vi "4031V2Project.vi"() -> ()   [LabVIEW 2024]
uses:
  <vilib>/Analysis/NI_AALBase.lvlib
  <vilib>/Utility/TradDaqScaling.llb/Convert Thermocouple Reading (array).vi
  <vilib>/Utility/file.llb/Write Delimited Spreadsheet (DBL).vi
  <vilib>/Utility/file.llb/Write Delimited Spreadsheet (string).vi
panel:
  out "Hot side Delta":dbl format="%#_13g"
  out "Cold Side Delta":dbl format="%#_13g"
  in  "Thermocouple Type":u16(ring)=2 items=["B", "E", "K", "K", "R", "S", "T", "N"]
  in  "Sampling rate":dbl
  in  "Number of Samples":dbl
  out "Tco Std":dbl
  out "Tco Mean":dbl
  out "Tci Std":dbl
  out "Tci Mean":dbl
  out "Tho SD 2":dbl
  out "Tho mean":dbl
  out "Thi SD":dbl
  out "Thi mean":dbl
  out "Cold Out":sgl[](graph)
  out "Cold In":sgl[](graph)
  out "Hot Out":sgl[](graph)
  out "Hot in":sgl[](graph)
  in  "?":bool
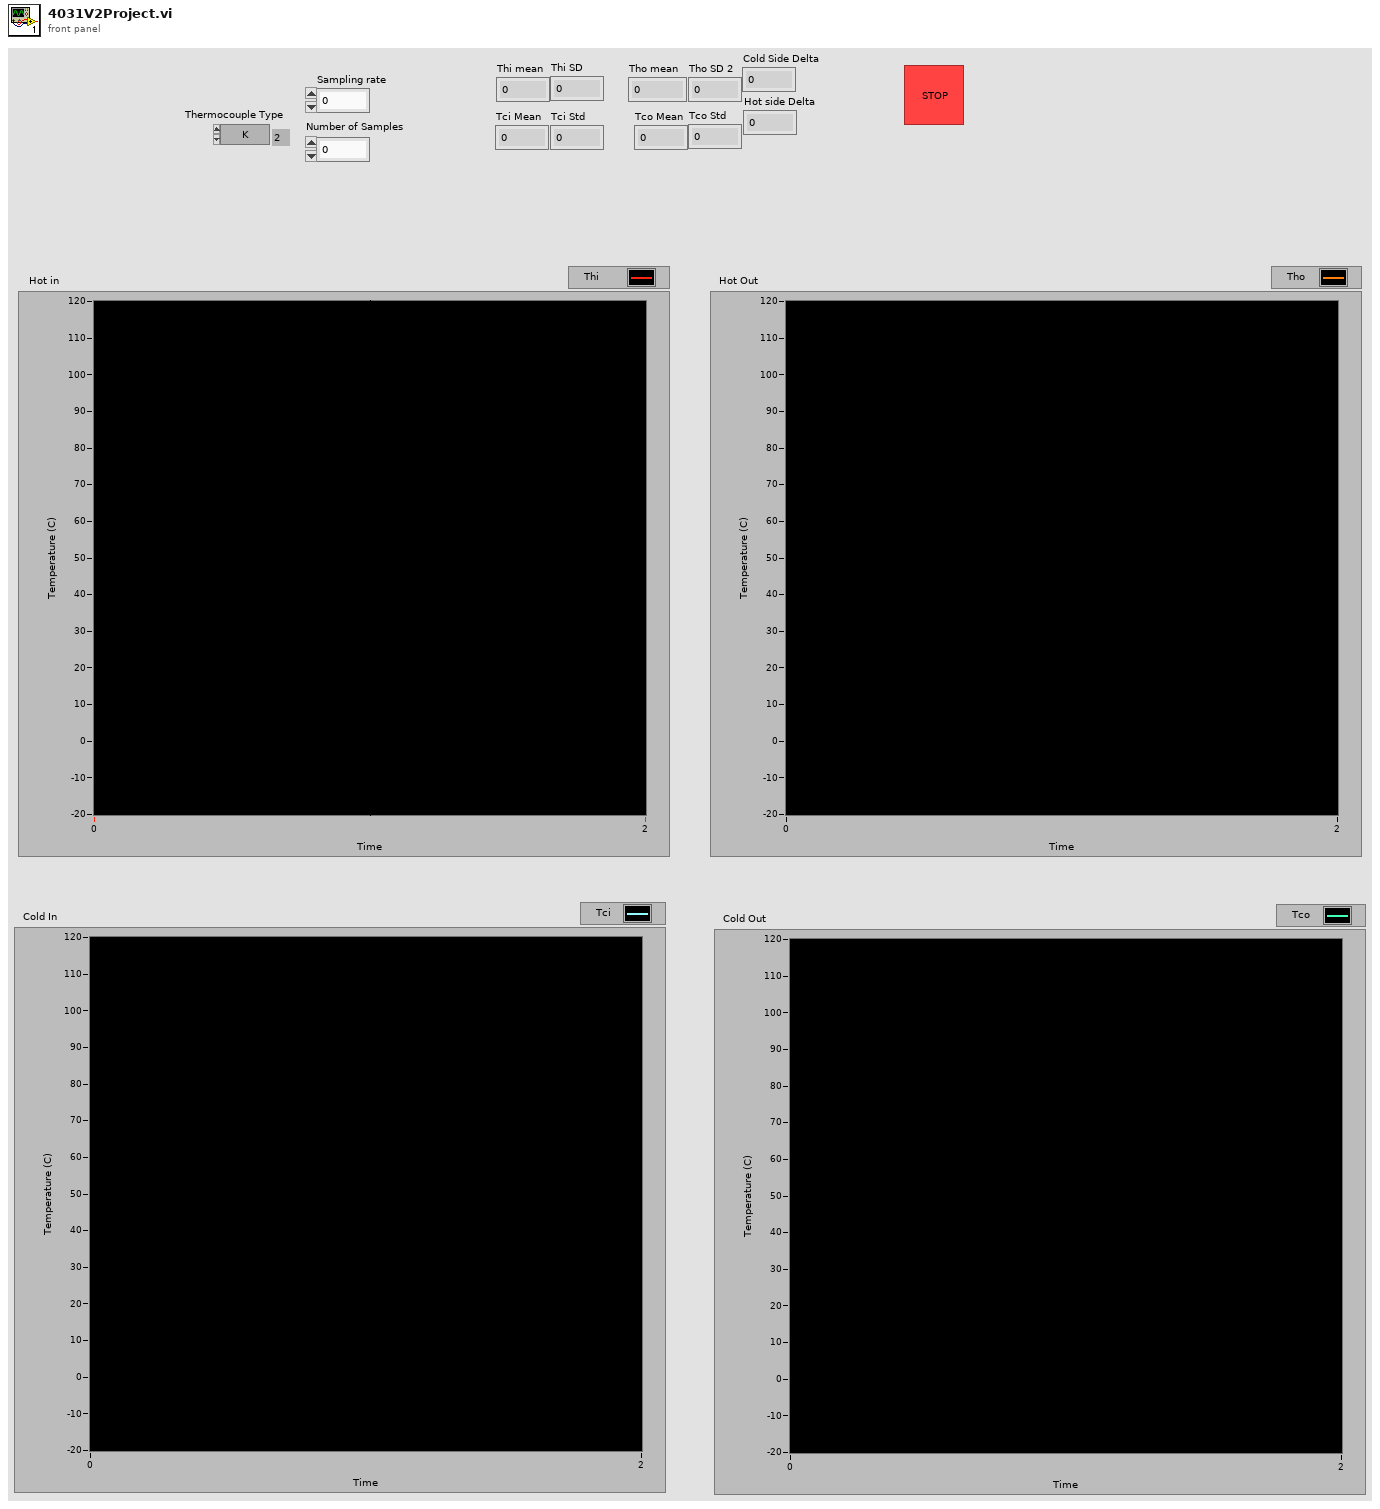
[diagram p1: front panel]
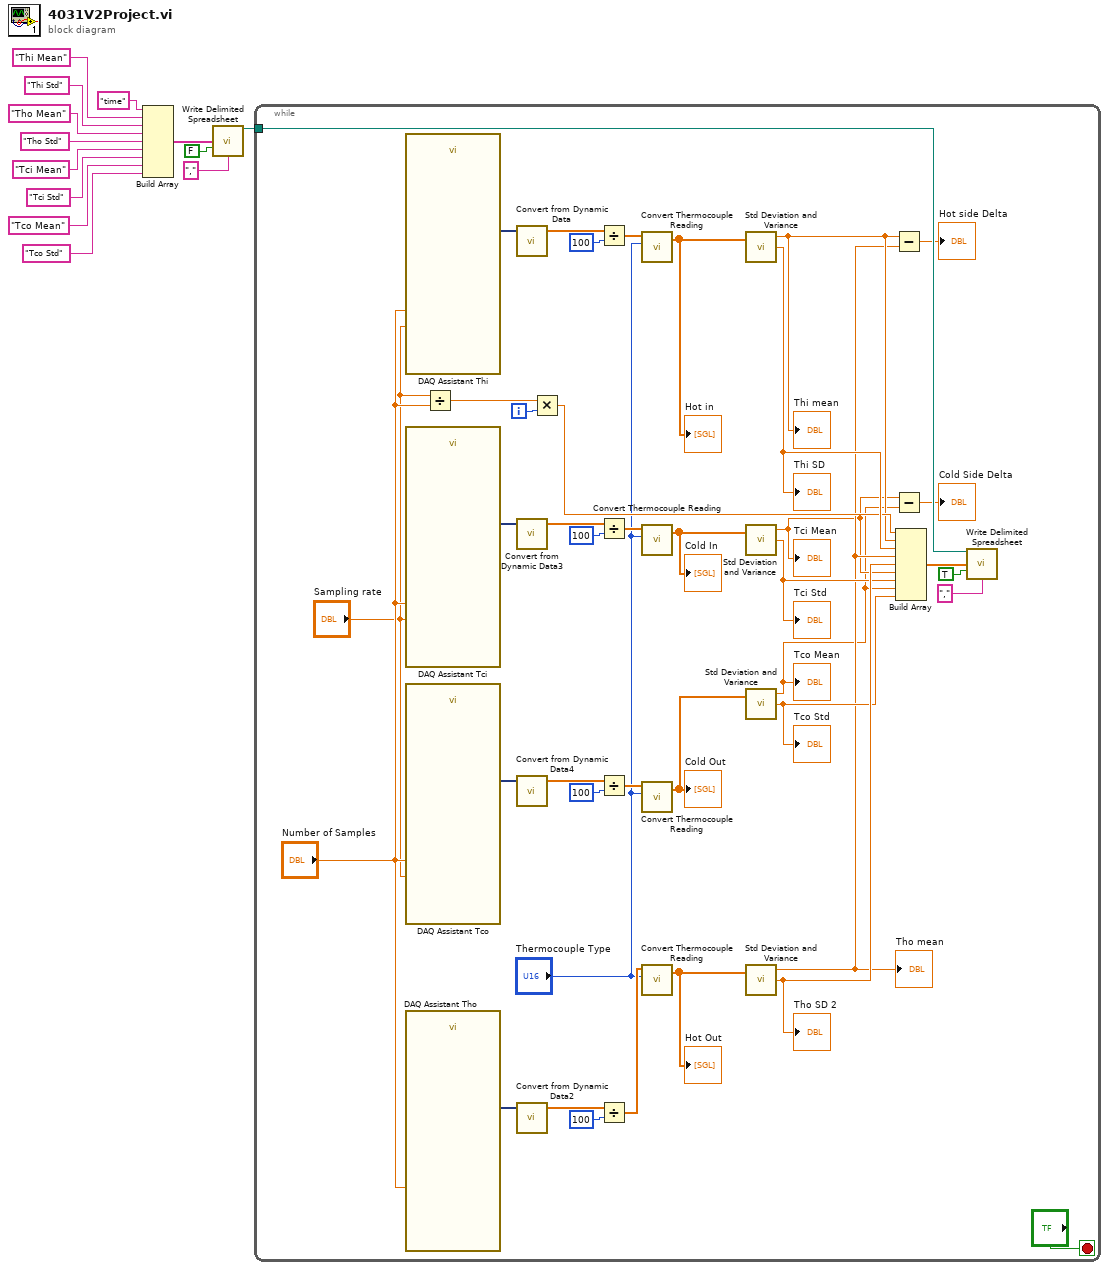
[diagram p0: block diagram]
diagram:
  n1 = Build Array("time", "Thi Mean", "Thi Std", "Tho Mean", "Tho Std", "Tci Mean", "Tci Std", "Tco Mean", "Tco Std") -> (w9:string[])
  n2 = call-poly <vilib>:"Write Delimited Spreadsheet.vi"("1D data"=w9, "append to file? (new file:F)"=FALSE, "delimiter (\\t)"=",") -> ("new file path (Not A Path if cancelled)"=w7:path)  [unwired: 11 in, 1 out]
  n3 = while {
    tunnel: w7 -> [w50]
    i -> [w36]
    stop <- "?" stop-if-true
    n4 = call "DAQ Assistant Thi"("rate"="Sampling rate", "number of samples"="Number of Samples") -> ("data"=w45:dynamicdata)  [unwired: 15 in, 2 out]
    n5 = call "DAQ Assistant Tci"("rate"="Sampling rate", "number of samples"="Number of Samples") -> ("data"=w35:dynamicdata)  [unwired: 15 in, 2 out]
    n6 = call "DAQ Assistant Tco"("rate"="Sampling rate", "number of samples"="Number of Samples") -> ("data"=w33:dynamicdata)  [unwired: 15 in, 2 out]
    n7 = call "DAQ Assistant Tho"("number of samples"="Number of Samples") -> ("data"=w41:dynamicdata)  [unwired: 16 in, 2 out]
    n8 = Divide(x="Sampling rate", y="Number of Samples") -> (x/y=w46:dbl)
    n9 = call "Convert from Dynamic Data"("Dynamic Data Type"=w45) -> ("Array"=w48:dbl[])  [unwired: 3 in]
    n10 = call "Convert from Dynamic Data3"("Dynamic Data Type"=w35) -> ("Array"=w34:dbl[])  [unwired: 3 in]
    n11 = call "Convert from Dynamic Data4"("Dynamic Data Type"=w33) -> ("Array"=w32:dbl[])  [unwired: 3 in]
    n12 = call "Convert from Dynamic Data2"("Dynamic Data Type"=w41) -> ("Array"=w43:dbl[])  [unwired: 3 in]
    n13 = Multiply(x=w46, y=w36) -> (x*y=w30:dbl)
    n14 = Divide(x=w48, y=100) -> (x/y=w47:dbl[])
    n15 = Divide(x=w34, y=100) -> (x/y=w39:dbl[])
    n16 = Divide(x=w32, y=100) -> (x/y=w37:dbl[])
    n17 = Divide(x=w43, y=100) -> (x/y=w42:dbl[])
    n18 = call-poly <vilib>:"Convert Thermocouple Reading.vi"("ThermocoupleType"="Thermocouple Type", "Voltage Array"=w47) -> ("Temperature Array"=w23:sgl[])  [unwired: 5 in]
    "Hot in" <- w23
    n19 = call-poly <vilib>:"Convert Thermocouple Reading.vi"("ThermocoupleType"="Thermocouple Type", "Voltage Array"=w39) -> ("Temperature Array"=w21:sgl[])  [unwired: 5 in]
    "Cold In" <- w21
    n20 = call-poly <vilib>:"Convert Thermocouple Reading.vi"("ThermocoupleType"="Thermocouple Type", "Voltage Array"=w37) -> ("Temperature Array"=w20:sgl[])  [unwired: 5 in]
    "Cold Out" <- w20
    n21 = call-poly <vilib>:"Convert Thermocouple Reading.vi"("ThermocoupleType"="Thermocouple Type", "Voltage Array"=w42) -> ("Temperature Array"=w22:sgl[])  [unwired: 5 in]
    "Hot Out" <- w22
    n22 = call <vilib>:"Std Deviation and Variance.vi"("X"=w23) -> ("mean"=w17:dbl, "standard deviation"=w31:dbl)  [unwired: 1 in, 1 out]
    "Thi mean" <- w17
    "Thi SD" <- w31
    n23 = call <vilib>:"Std Deviation and Variance.vi"("X"=w21) -> ("mean"=w15:dbl, "standard deviation"=w28:dbl)  [unwired: 1 in, 1 out]
    "Tci Mean" <- w15
    "Tci Std" <- w28
    n24 = call <vilib>:"Std Deviation and Variance.vi"("X"=w20) -> ("mean"=w14:dbl, "standard deviation"=w27:dbl)  [unwired: 1 in, 1 out]
    "Tco Mean" <- w14
    "Tco Std" <- w27
    n25 = call <vilib>:"Std Deviation and Variance.vi"("X"=w22) -> ("mean"=w16:dbl, "standard deviation"=w29:dbl)  [unwired: 1 in, 1 out]
    "Tho mean" <- w16
    "Tho SD 2" <- w29
    n26 = Subtract(x=w17, y=w16) -> (x-y=→"Hot side Delta":dbl)
    n27 = Subtract(x=w15, y=w14) -> (x-y=→"Cold Side Delta":dbl)
    n28 = Build Array(w30, w17, w31, w16, w29, w15, w28, w14, w27) -> (w52:dbl[])
    n29 = call-poly <vilib>:"Write Delimited Spreadsheet.vi"("file path (dialog if empty)"=w50, "1D data"=w52, "append to file? (new file:F)"=TRUE, "delimiter (\\t)"=",") -> ()  [unwired: 10 in, 2 out]
  }
